vi "UartTest.vi"() -> ()   [LabVIEW 2019]
uses:
  <vilib>/myRIO/Instrument Drivers/Onboard IO/UART/typedef/VISA Configuration.ctl
  <vilib>/Instr/_visa.llb/VISA Configure Serial Port (Instr).vi
  <vilib>/myRIO/Express VI/Onboard IO/UART/UART Express VI.xnode
  <vilib>/myRIO/Instrument Drivers/Onboard IO/UART/UART.lvlib
panel:
  out "Read":string
  in  "Write":string
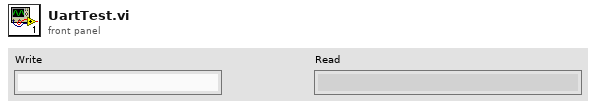
[diagram p1: front panel]
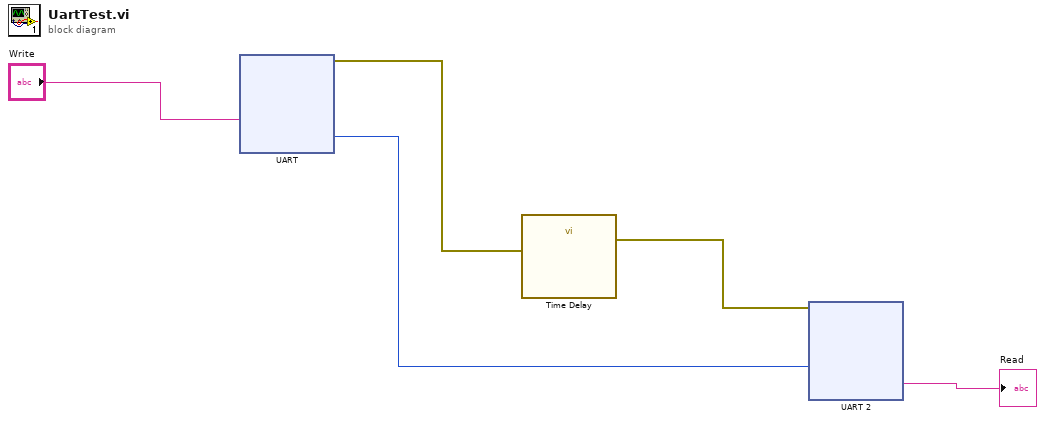
[diagram p0: block diagram]
diagram:
  n1 = xnode "UART"("Characters to Write"="Write") -> ("Character Count"=w1:u32, "error out"=w3:errorcluster)  [unwired: 1 in]
  n2 = call "Time Delay"("error in (no error)"=w3) -> ("error out"=w2:errorcluster)  [unwired: 10 in]
  n3 = xnode "UART 2"("Character Count"=w1, "error in (no error)"=w2) -> ("Characters Read"=→"Read":string)  [unwired: 1 out]
